vi "calibrationSpectrometer_getSample_SpectTemperature.vi"(8 "error in (no error)":errorcluster, 11 "SpectTemperature_Ctl":T1) -> (0 "error out":errorcluster, 2 "function return":i32, 3 "SpectTemperature_Ctl out":T1)   [LabVIEW 2016, in "SALLV_calibrationSpectrometer.lvlib"]
doc: "int calibrationSpectrometer_shm_getSample_SpectTemperatureLV(calibrationSpectrometer_SpectTemperatureLV *SpectTemperature_Ctl );"
uses:
  SALLV_calibrationSpectrometer.lvlib
  DataTypes/SpectTemperature.ctl
  SALLV_calibrationSpectrometer.so
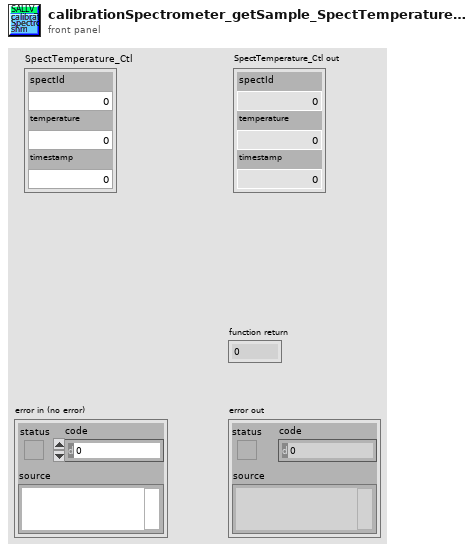
[diagram p1: front panel]
types:
  T1 = typedef "SALLV_calibrationSpectrometer.lvlib/SpectTemperature.ctl" = cluster{"spectId":u16, "temperature":dbl, "timestamp":dbl}
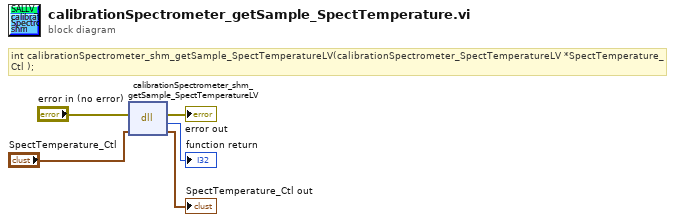
[diagram p0: block diagram]
diagram:
  # "int calibrationSpectrometer_shm_getSample_SpectTemperatureLV(calibrationSpectrometer_SpectTemperatureLV *SpectTemperature_Ctl );"
  n1 = dll-call lib="home/harini/TCS/sallv_sedspectrometer/SALLV_calibrationSpectrometer.*" fn="calibrationSpectrometer_shm_getSample_SpectTemperatureLV"(error in="error in (no error)", "SpectTemperature_Ctl"="SpectTemperature_Ctl") -> (error out=→"error out":errorcluster, →"function return":i32, "SpectTemperature_Ctl"=→"SpectTemperature_Ctl out":T1)  [unwired: 2 in, 1 out]
